vi "DAQ Read Analog Input.vi"(8 "error in":errorcluster, 11 "task/channels in":refnum<k21>) -> (0 "error out":errorcluster, 2 "Voltage":dbl format="%0.2f", 3 "task out":refnum<k21>)   [LabVIEW 2021]
uses:
  <vilib>/DAQmx/read.llb/DAQmx Read (Analog DBL 1Chan 1Samp).vi
  <vilib>/DAQmx/miscellaneous.llb/DAQmx Fill In Error Info.vi
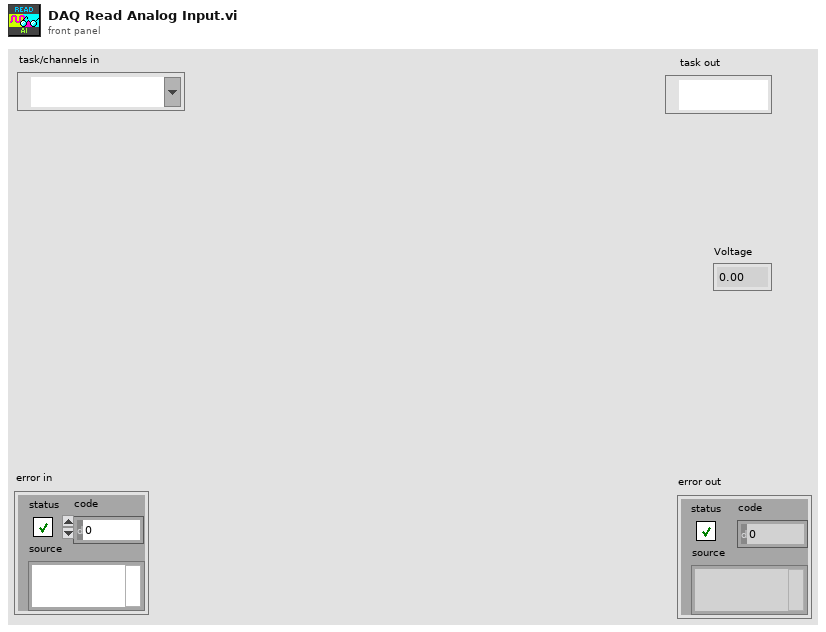
[diagram p1: front panel]
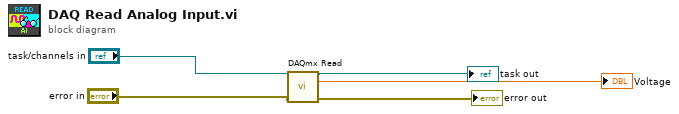
[diagram p0: block diagram]
diagram:
  n1 = call-poly <vilib>:"DAQmx Read.vi"("task/channels in"="task/channels in", "error in"="error in") -> ("task out"=→"task out":refnum<k21>, "data"=→"Voltage":dbl, "error out"=→"error out":errorcluster)  [unwired: 11 in]
